vi "DiscCounter.vi"() -> ()   [LabVIEW 2012]
uses:
  Robot Global Data.vi
panel:
  out "Has Been False":bool
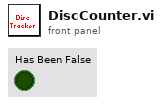
[diagram p1: front panel]
types:
  T1 = typedef "WPI_DigitalInputDevRef.ctl" = cluster{"DevStatus":errorcluster, "DIO Channel":T2, "Digital Module":T3}
  T2 = typedef "FPGA_DIOChannel.ctl" = enum8{"DIO 1", "DIO 2", "DIO 3", "DIO 4", "DIO 5", "DIO 6", "DIO 7", "DIO 8", "DIO 9", "DIO 10", "DIO 11", "DIO 12", "DIO 13", "DIO 14", "Invalid"}
  T3 = typedef "FPGA_TypedefDigitalModule.ctl" = enum16{"Digital Module 1", "Digital Module 2"}
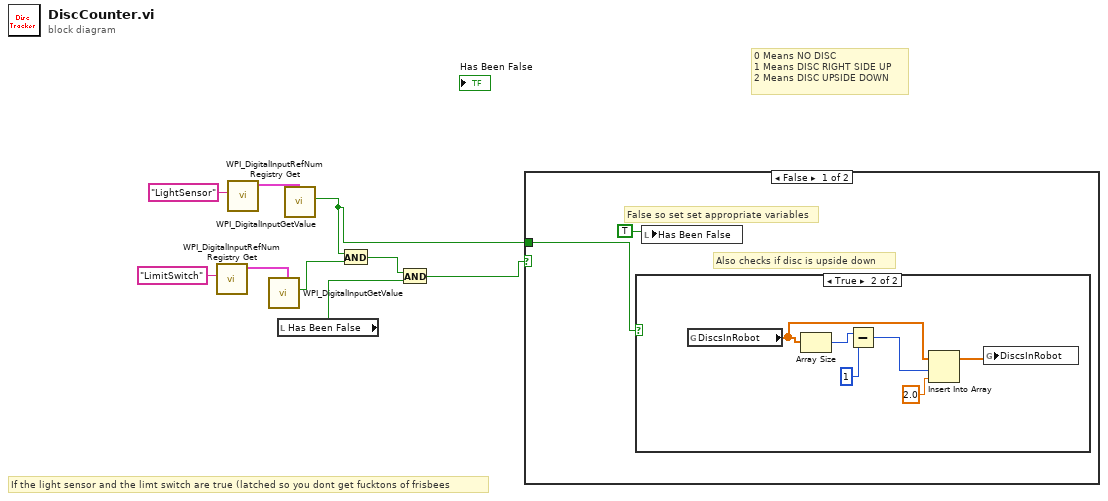
[diagram p0: block diagram]
diagram:
  # "0 Means NO DISC\n1 Means DISC RIGHT SIDE UP\n2 Means DISC UPSIDE DOWN"
  # "If the light sensor and the limt switch are true (latched so you dont get fucktons of frisbees"
  n1 = call <vilib>:"WPI_DigitalInputRefNum Registry Get.vi"("refnum name"="LimitSwitch") -> ("DigitalInputDevRef"=w6:T1)  [unwired: 9 in, 1 out]
  n2 = call <vilib>:"WPI_DigitalInputRefNum Registry Get.vi"("refnum name"="LightSensor") -> ("DigitalInputDevRef"=w9:T1)  [unwired: 9 in, 1 out]
  n3 = call <vilib>:"WPI_DigitalInputGetValue.vi"("DigitalInputDevRef"=w6) -> ("Value"=w2:bool)  [unwired: 8 in, 2 out]
  n4 = local read "Has Been False"() -> (w4:bool)
  n5 = call <vilib>:"WPI_DigitalInputGetValue.vi"("DigitalInputDevRef"=w9) -> ("Value"=w1:bool)  [unwired: 8 in, 2 out]
  n6 = And(x=w1, y=w2) -> (x .and. y?=w5:bool)
  n7 = And(x=w5, y=w4) -> (x .and. y?=w3:bool)
  n8 = case shown="False" w3 {
    tunnel: w1 -> [w10 _]
    frame False {
      # "Also checks if disc is upside down"
      # "False so set set appropriate variables"
      n9 = case shown="True" w10 {
        frame False {
        }
        frame True {
          n10 = global read "Robot Global Data.vi" "DiscsInRobot"() -> (w14:dbl[])
          n11 = Array Size(array=w14) -> (size(s)=w17:i32)
          n12 = Subtract(x=w17, y=1) -> (x-y=w15:i32)
          n13 = Insert Into Array(array=w14, index=w15, new element=2.0 ("new element/subarray")) -> (w12:dbl[])
          n14 = global write "Robot Global Data.vi" "DiscsInRobot"(w12) -> ()
        }
      }
      n15 = local write "Has Been False"(TRUE ("Has Been False")) -> ()
    }
    frame True {
      # "True so add disc to array"
    }
  }
